vi "Decide Whether To Pop-up New Error Dialogue.vi"(6 "Is New Error Dialogue GUI Running Already?":bool, 8 "Error In":errorcluster, 9 "Pop-up New Error Dialogue Setting (Default = Pop-up Dialogue)":T1, 10 "Newly Reported Error":T2, 11 "Module Data in":T4) -> (0 "Error Out":errorcluster)   [LabVIEW 2023, in "Error Manager.lvlib"]
doc: "This VI decides whether the \"New Error Dialogue\" should be popped-up (displayed) to the user.\n\nThe \"New Error Dialogue\" is popped-up if and only if all the following conditions are met:\n1. The \"Pop-up New Error Dialogue Setting\" is set to \"Pop-up New Error Dialogue\"\n2. The \"New Error Dialogue\" GUI is not already running (being displayed to the user)\n3. The newly reported error is indeed a \"New Error Code Error\" - meaning it is an error code that is not already found amongst the \"unread errors\"."
uses:
  Error Manager.lvlib
  Module Data (cluster).ctl
  Handled Error (cluster).ctl
  Read-Unread Status (enum).ctl
  Display Order (enum).ctl
  Error in current one-second interval (cluster).ctl
  Reported Error (cluster).ctl
  Public API VIs/Pop-up New Error Dialogue Instruction (enum).ctl
  Public API VIs/Pop-up New Error Dialogue Setting (enum).ctl
panel:
  out "Pop-up \"New Error Dialogue\" GUI?":bool
  out "Same Error Code found amongst the \"unread errors\"?":bool
  out "New Error Code?":bool
  # "Development\nControls or indicators that are useful for development or testing, but which are not outputs of the VI."
  # "Input\nInputs to the VI"
  # "Output\nOutputs of the VI"
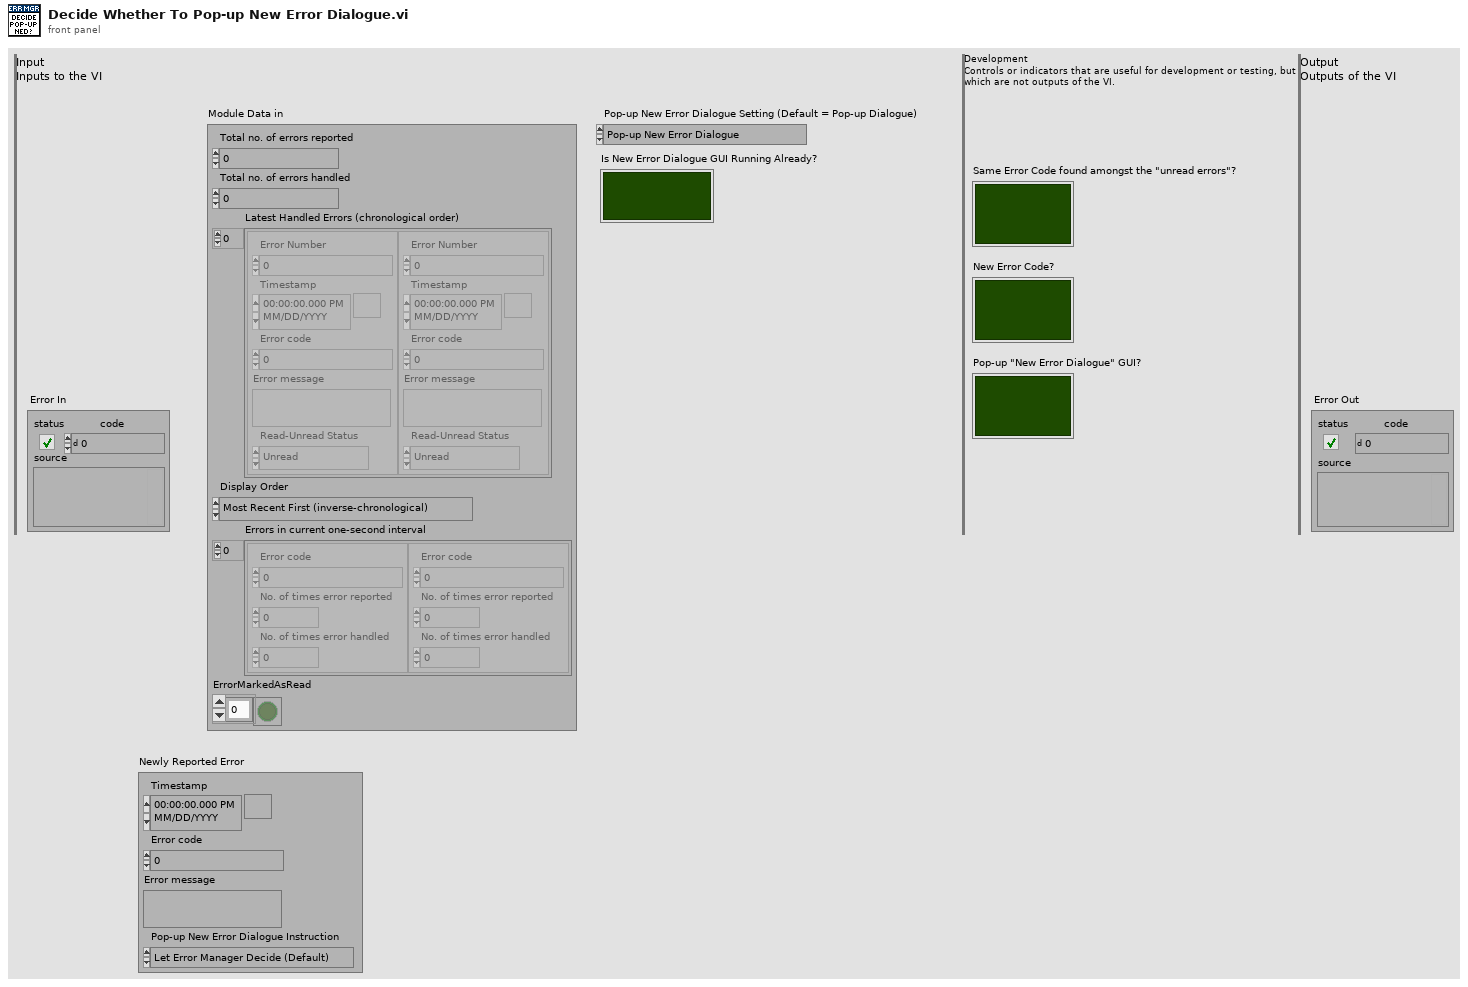
[diagram p1: front panel]
types:
  T1 = typedef "Error Manager.lvlib/Pop-up New Error Dialogue Setting (enum).ctl" = enum16{"Pop-up New Error Dialogue", "Don't pop-up New Error Dialogue"}
  T2 = typedef "Error Manager.lvlib/Reported Error (cluster).ctl" = cluster{"Timestamp":timestamp, "Error code":i32, "Error message":string, "Pop-up New Error Dialogue Instruction":T3}
  T3 = typedef "Error Manager.lvlib/Pop-up New Error Dialogue Instruction (enum).ctl" = enum16{"Let Error Manager Decide (Default)", "Don't pop-up", "Pop-up"}
  T4 = typedef "Error Manager.lvlib/Module Data (cluster).ctl" = cluster{"Total no. of errors reported":i32, "Total no. of errors handled":i32, "Latest Handled Errors (chronological order)":T5[], "Display Order":T7, "Errors in current one-second interval":T8[], "ErrorMarkedAsRead":bool[]}
  T5 = typedef "Error Manager.lvlib/Handled Error (cluster).ctl" = cluster{"Error Number":i32, "Timestamp":timestamp, "Error code":i32, "Error message":string, "Read-Unread Status":T6}
  T6 = typedef "Error Manager.lvlib/Read-Unread Status (enum).ctl" = enum16{"Unread", "Read"}
  T7 = typedef "Error Manager.lvlib/Display Order (enum).ctl" = enum16{"Most Recent First (inverse-chronological)", "Oldest First (chronological)"}
  T8 = typedef "Error Manager.lvlib/Error in current one-second interval (cluster).ctl" = cluster{"Error code":i32, "No. of times error reported":u32, "No. of times error handled":u32}
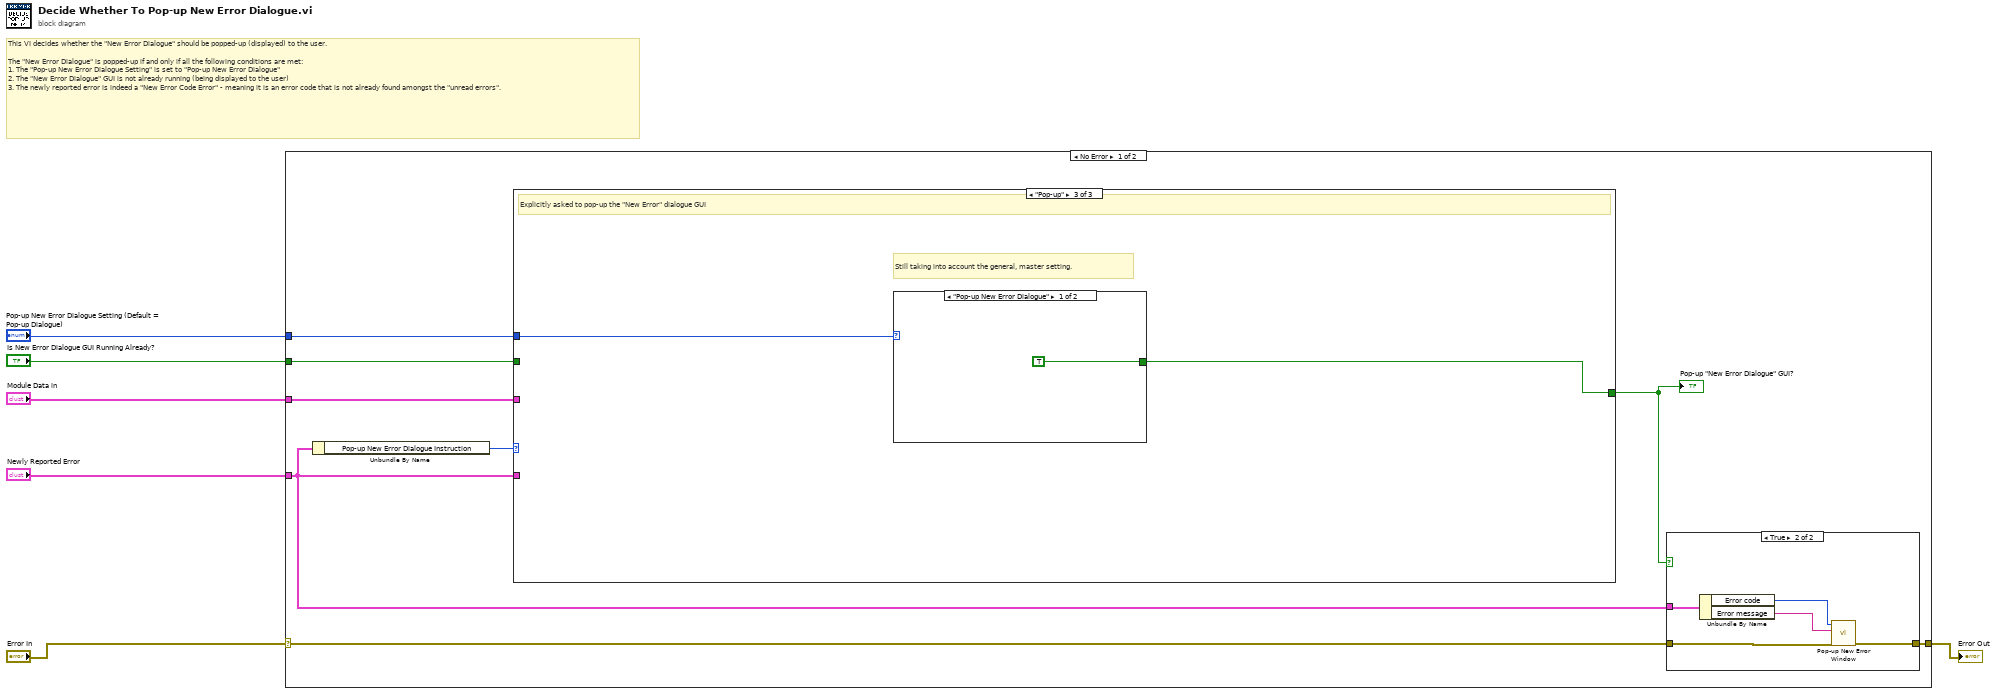
[diagram p0: block diagram]
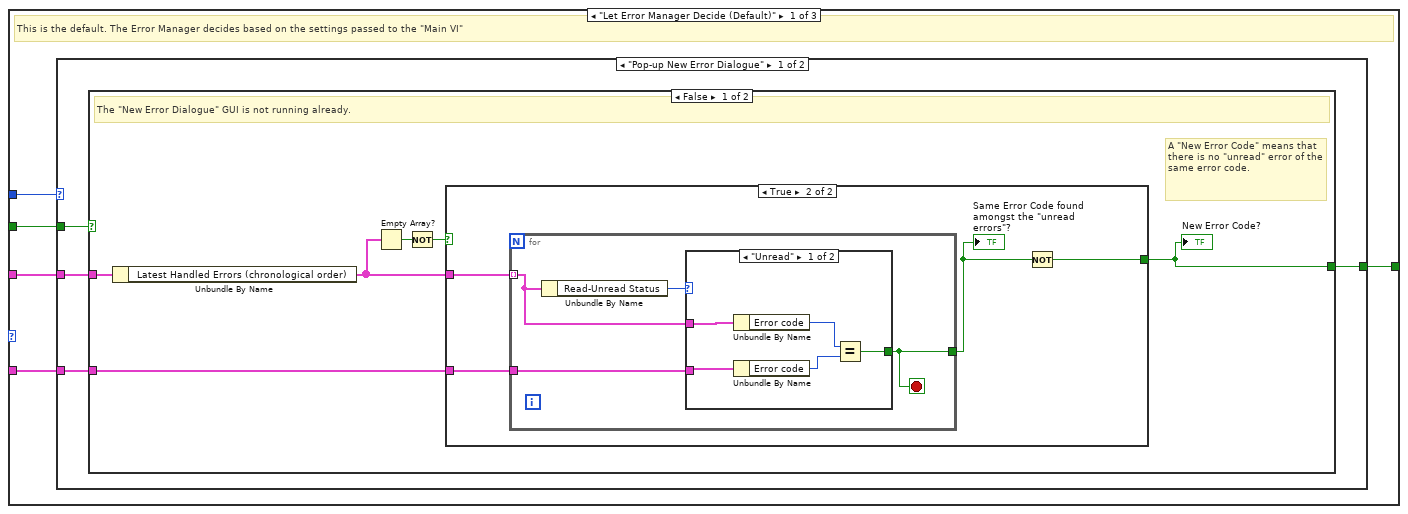
[diagram p2: hidden frame]
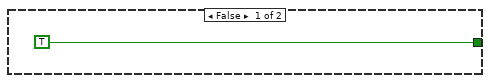
[diagram p3: hidden frame]
diagram:
  # "This VI decides whether the \"New Error Dialogue\" should be popped-up (displayed) to the user.\n\nThe \"New Error Dialogue\" is popped-up if and only if all the following conditions are met:\n1. The \"Pop-up New Error Dialogue Setting\" is set to \"Pop-up New Error Dialogue\"\n2. The \"New Error Dialogue\" GUI is not already running (being displayed to the user)\n3. The newly reported error is indeed a \"New Error Code Error\" - meaning it is an error code that is not already found amongst the \"unread errors\"."
  n1 = case shown="No Error" "Error In" {
    selector: "Error In" -> [w11 w53]
    tunnel: [w10 w53] -> w5
    tunnel: "Module Data in" -> [w14 _]
    tunnel: "Newly Reported Error" -> [w8 _]
    tunnel: "Is New Error Dialogue GUI Running Already?" -> [w13 _]
    tunnel: "Pop-up New Error Dialogue Setting (Default = Pop-up Dialogue)" -> [w12 _]
    frame No Error {
      n2 = Unbundle By Name(w8) -> ("Pop-up New Error Dialogue Instruction"=w7:T3)
      n3 = case shown="\"Pop-up\"" w7 {
        tunnel: w14 -> [w19 _ _]
        tunnel: w13 -> [w18 _ _]
        tunnel: w12 -> [w17 _ w45]
        tunnel: [w16 _ w44] -> w9
        tunnel: w8 -> [w15 _ _]
        frame "Let Error Manager Decide (Default)" {
          # "This is the default. The Error Manager decides based on the settings passed to the \"Main VI\""
          n4 = case shown="\"Pop-up New Error Dialogue\"" w17 {
            tunnel: w19 -> [w23 _]
            tunnel: w15 -> [w22 _]
            tunnel: w18 -> [w21 _]
            tunnel: [w20 _] -> w16
            frame "Pop-up New Error Dialogue" {
              n5 = case shown="False" w21 {
                tunnel: w23 -> [w29 _]
                tunnel: w22 -> [w25 _]
                tunnel: [w24 _] -> w20
                frame False {
                  # "A \"New Error Code\" means that there is no \"unread\" error of the same error code."
                  # "The \"New Error Dialogue\" GUI is not running already."
                  n6 = Unbundle By Name(w29) -> ("Latest Handled Errors (chronological order)"=w26:T5[])
                  n7 = Empty Array?(array=w26) -> (empty?=w28:bool)
                  n8 = Not(x=w28) -> (.not. x?=w27:bool)
                  n9 = case shown="True" w27 {
                    tunnel: [TRUE w32] -> w24
                    tunnel: w26 -> [_ w34]
                    tunnel: w25 -> [_ w33]
                    frame False {
                    }
                    frame True {
                      n10 = for {
                        tunnel: w34 -> [w36] mode=indexing
                        tunnel: w33 -> [w37]
                        tunnel: [w35] -> w31
                        stop <- w35 stop-if-true
                        n11 = Unbundle By Name(w36) -> ("Read-Unread Status"=w38:T6)
                        n12 = case shown="\"Unread\"" w38 {
                          tunnel: w37 -> [w42 _]
                          tunnel: w36 -> [w43 _]
                          tunnel: [w39 _] -> w35
                          frame "Unread" {
                            n13 = Unbundle By Name(w43) -> ("Error code"=w41:i32)
                            n14 = Unbundle By Name(w42) -> ("Error code"=w40:i32)
                            n15 = Equal?(x=w41, y=w40) -> (x = y?=w39:bool)
                          }
                          frame "Read" {
                          }
                        }
                      }
                      "Same Error Code found amongst the \"unread errors\"?" <- w31
                      n16 = Not(x=w31) -> (.not. x?=w32:bool)
                    }
                  }
                  "New Error Code?" <- w24
                }
                frame True {
                  # "Do not enqueue a message to pop-up the GUI again. Otherwise, could lead to a cycle of GUIs being popped-up more quickly than the user can close them. Not desired."
                  # "The \"New Error Dialogue\" GUI is running already."
                }
              }
            }
            frame "Don't pop-up New Error Dialogue" {
            }
          }
        }
        frame "Don't pop-up" {
          # "Explicitly asked NOT TO pop-up the \"New Error\" dialogue GUI"
        }
        frame "Pop-up" {
          # "Still taking into account the general, master setting."
          # "Explicitly asked to pop-up the \"New Error\" dialogue GUI"
          n17 = case shown="\"Pop-up New Error Dialogue\"" w45 {
            tunnel: [TRUE _] -> w44
            frame "Pop-up New Error Dialogue" {
            }
            frame "Don't pop-up New Error Dialogue" {
              # "The general, master setting explictly forbids the dialogue from being popped, and has precedence over explicitly requesting an individual error to be popped-up (the per-error instruction)."
            }
          }
        }
      }
      "Pop-up \"New Error Dialogue\" GUI?" <- w9
      n18 = case shown="True" w9 {
        tunnel: w11 -> [w47 w52]
        tunnel: [w47 w51] -> w10
        tunnel: w8 -> [_ w50]
        frame False {
        }
        frame True {
          n19 = Unbundle By Name(w50) -> ("Error code"=w49:i32, "Error message"=w48:string)
          n20 = call "Pop-up New Error Window.vi"("Error In"=w52, "Error Message"=w48, "Error Code"=w49) -> ("Error Out"=w51:errorcluster)  [unwired: 8 in]
        }
      }
    }
    frame Error {
    }
  }
  "Error Out" <- w5
